vi "set_stopThread.vi"(0 "HGF_ThreadWorker":refnum<class "HGF_ThreadWorker.lvclass">, 2 "stopThread (T)":bool=TRUE, 5 "error in (no error)":errorcluster) -> (14 "dup HGF_ThreadWorker":refnum<class "HGF_ThreadWorker.lvclass">, 19 "error out":errorcluster)   [LabVIEW 2014, in "HGF_BaseClasses.lvlib" / "HGF_ThreadWorker.lvclass"]
doc: "Set flag to stop thread."
uses:
  HGF_ThreadWorker.lvclass
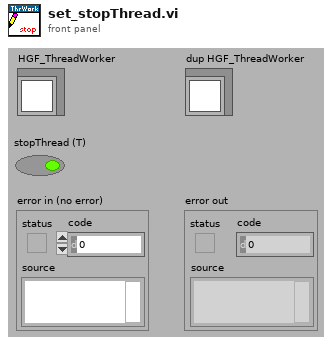
[diagram p1: front panel]
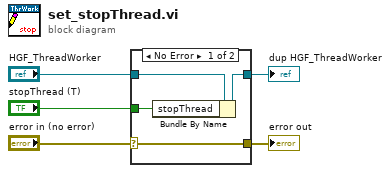
[diagram p0: block diagram]
diagram:
  n1 = case shown="No Error" "error in (no error)" {
    selector: "error in (no error)" -> [w9 w10]
    tunnel: [w9 w10] -> w4
    tunnel: [w8 w11] -> w2
    tunnel: "HGF_ThreadWorker" -> [w6 w11]
    tunnel: "stopThread (T)" -> [w7 _]
    frame No Error {
      n2 = Bundle By Name(cluster=w6, "stopThread"=w7) -> (w8:refnum<class "HGF_ThreadWorker.lvclass">)
    }
    frame Error {
    }
  }
  "error out" <- w4
  "dup HGF_ThreadWorker" <- w2
